vi "export_excel.vi"(6 "table":string[][](array[string]), 7 "position (excel).row":i32, 8 "error in (no error)":errorcluster, 9 "template_filename":string, 10 "result_filename":string, 11 "position (excel).column":i32) -> (0 "error out":errorcluster)   [LabVIEW 2017]
uses:
  <vilib>/Utility/NIReport.llb/Append Text Table to Report (wrap).vi
  <vilib>/Utility/NIReport.llb/NI_report.lvclass
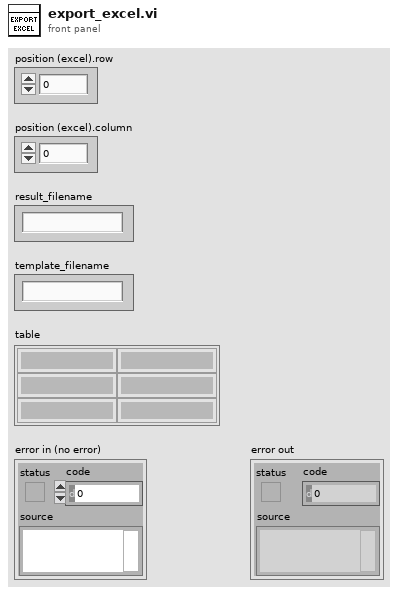
[diagram p1: front panel]
types:
  T1 = cluster{"position (excel)":cluster{"row":i32, "column":i32}, "name (excel)":string, "bookmark (word)":string}
  T2 = enum16{"maximized", "minimized", "normal", "no change"}
  T3 = enum16{"Standard Report", "HTML", "Word", "Excel"}
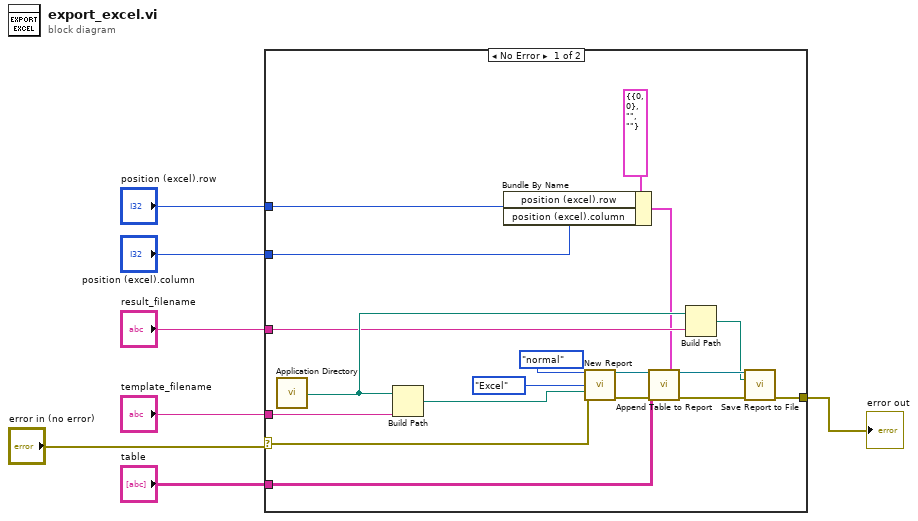
[diagram p0: block diagram]
diagram:
  n1 = case shown="No Error" "error in (no error)" {
    selector: "error in (no error)" -> [w9 w26]
    tunnel: "table" -> [w16 _]
    tunnel: "template_filename" -> [w14 _]
    tunnel: "position (excel).row" -> [w13 _]
    tunnel: "position (excel).column" -> [w12 _]
    tunnel: "result_filename" -> [w11 _]
    tunnel: [w10 w26] -> w6
    frame No Error {
      n2 = call <vilib>:"Application Directory.vi"() -> ("Application Directory"=w18:path)
      n3 = Build Path(base path=w18, name or relative path=w14) -> (appended path=w23:path)
      n4 = Bundle By Name(cluster=T1 {"position (excel)"={"row"=0, "column"=0}, "name (excel)"="", "bookmark (word)"=""} ("MS Office parameters"), "position (excel).row"=w13, "position (excel).column"=w12) -> (w8:T1)
      n5 = call <vilib>:"New Report.vi"("window state (normal)"=T2."normal", "report type"=T3."Excel", "template (empty)"=w23, "error in (no error)"=w9) -> ("report out"=w22:refnum<class "NI_report.lvclass">, "error out"=w20:errorcluster)  [unwired: 10 in]
      n6 = call-poly <vilib>:"Append Table to Report.vi"("report in"=w22, "MS Office parameters"=w8, "text data"=w16, "error in (no error)"=w20) -> ("report out"=w21:refnum<class "NI_report.lvclass">, "error out"=w19:errorcluster)  [unwired: 8 in, 2 out]
      n7 = Build Path(base path=w18, name or relative path=w11) -> (appended path=w17:path)
      n8 = call-dynamic "Save Report to File.vi"("report in"=w21, "report file path"=w17, "error in (no error)"=w19) -> ("error out"=w10:errorcluster)  [unwired: 11 in, 1 out]
    }
    frame Error {
    }
  }
  "error out" <- w6
